vi "Initialize Components.vi"(7 "Components":refnum<class "Component.lvclass">[](array[class]), 8 "error in (no error)":errorcluster, 10 "Plugin Configuration":refnum<class "Plugin Configuration.lvclass">, 11 "Transceiver Thread in":refnum<class "Transceiver Thread.lvclass">) -> (0 "error out":errorcluster, 3 "Transceiver Thread out":refnum<class "Transceiver Thread.lvclass">)   [LabVIEW 2020, in "DSF Core.lvlib" / "Transceiver Thread.lvclass"]
uses:
  Transceiver Thread.lvclass
  Component/Component.lvclass
  Configuration/Core/Plugin/Plugin Configuration.lvclass
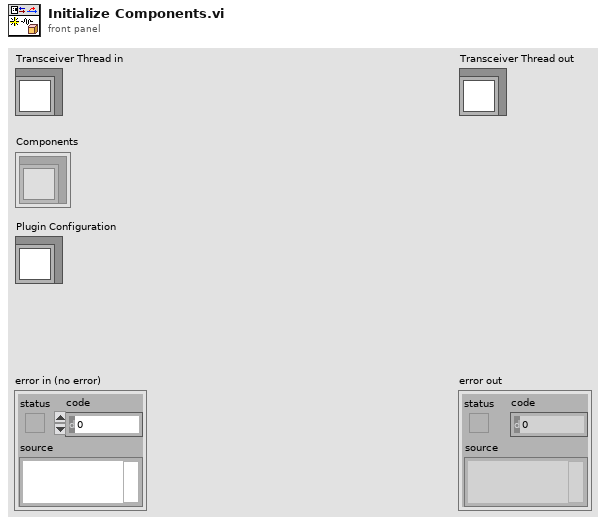
[diagram p1: front panel]
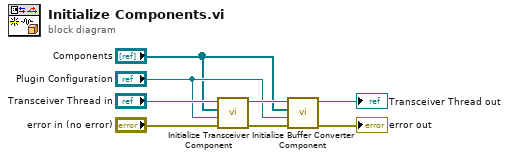
[diagram p0: block diagram]
diagram:
  n1 = call "Initialize Transceiver Component.vi"("error in (no error)"="error in (no error)", "Plugin Configuration"="Plugin Configuration", "Components"="Components", "Transceiver Thread in"="Transceiver Thread in") -> ("error out"=w6:errorcluster, "Transceiver Thread out"=w5:refnum<class "Transceiver Thread.lvclass">)  [unwired: 6 in]
  n2 = call "Initialize Buffer Converter Component.vi"("error in (no error)"=w6, "Plugin Configuration"="Plugin Configuration", "Components"="Components", "Transceiver Thread in"=w5) -> ("error out"=→"error out":errorcluster, "Transceiver Thread out"=→"Transceiver Thread out":refnum<class "Transceiver Thread.lvclass">)  [unwired: 6 in]
